vi "Get Array Element Offsets.vi"(8 "error in (no error)":errorcluster, 9 "Max Index":i32=2147483647, 10 "Offset":i32, 11 "JSON":string="[1,2,3]") -> (0 "error out":errorcluster, 1 "Elements":T1[](array[typedef]), 2 "Offset past Array":i32, 4 "Comma Needed for Insert":bool)   [LabVIEW 2024, in "JSONtext.lvlib"]
uses:
  JSONtext.lvlib
  Found Items.ctl
  Parsing State.ctl
  Comma Needed for Insert.ctl
  Advance past Line Ending.vi
  Advance past String.vi
  Advance past Number.vi
  Advance past Array.vi
  Advance past Object.vi
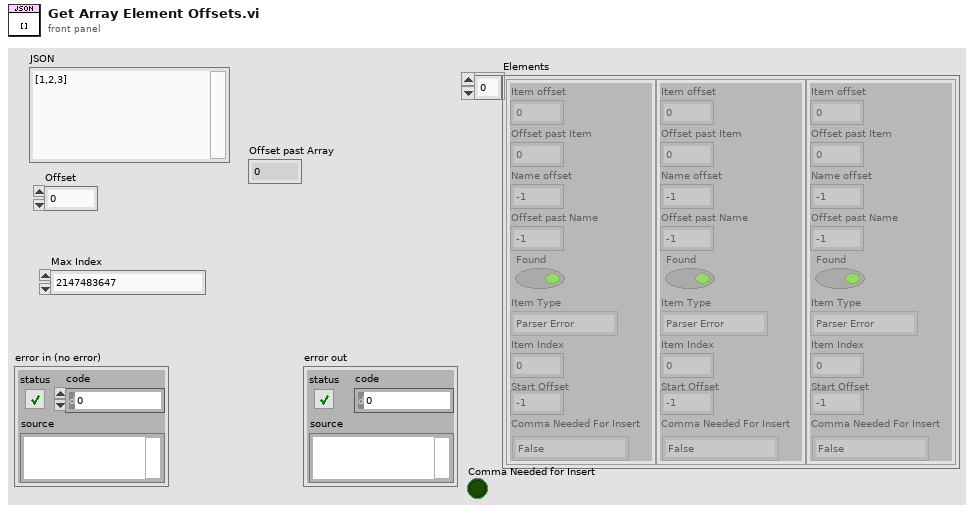
[diagram p1: front panel]
types:
  T1 = typedef "JSONtext.lvlib/Found Items.ctl" = cluster{"Item offset":i32, "Offset past Item":i32, "Name offset":i32, "Offset past Name":i32, "Found":bool, "Item Type":T2, "Item Index":i32, "Start Offset":i32, "Comma Needed For Insert":T3}
  T2 = typedef "JSONtext.lvlib/Parsing State.ctl" = enum16{"Parser Error", "Object", "Array", "String", "Number/Other", "Leading Whitespace", "Object end", "Array end", "Value end"}
  T3 = typedef "JSONtext.lvlib/Comma Needed for Insert.ctl" = enum8{"False", "True", "Following"}
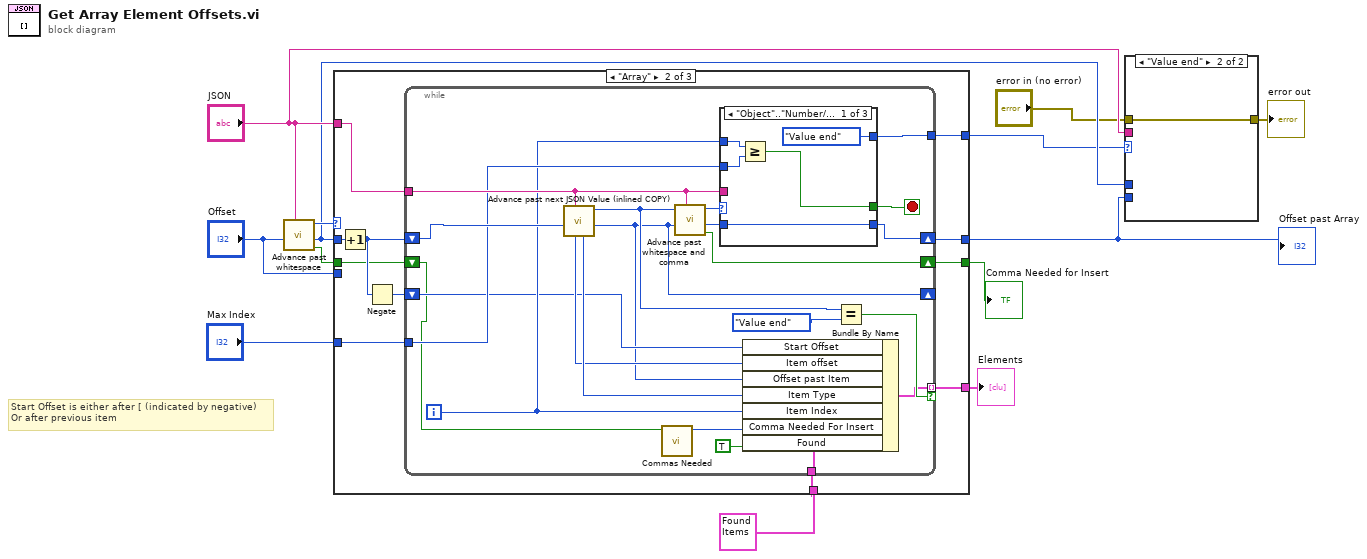
[diagram p0: block diagram]
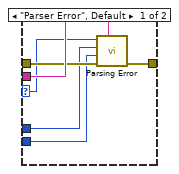
[diagram p2: hidden frame]
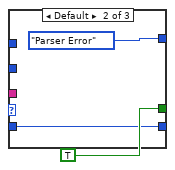
[diagram p4: hidden frame]
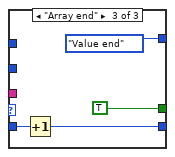
[diagram p5: hidden frame]
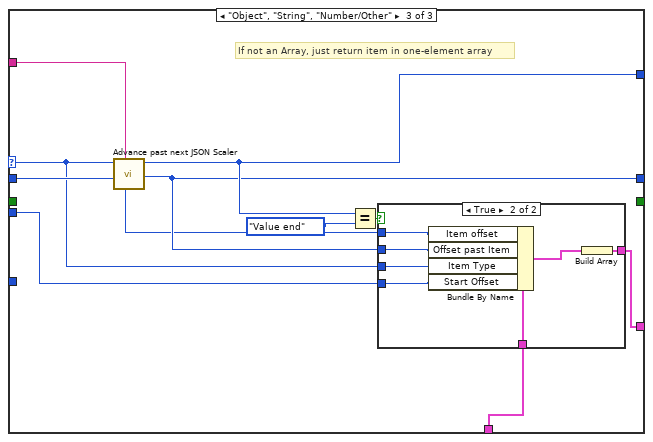
[diagram p6: hidden frame]
diagram:
  # "Start Offset is either after [ (indicated by negative)\nOr after previous item"
  n1 = call "Advance past whitespace.vi"("JSON"="JSON", "Offset"="Offset") -> ("Comma Not Found"=w2:bool, "Offset of first non-whitespace"=w11:i32, "Parser State"=w13:T2)  [unwired: 7 in]
  n2 = case shown="\"Array\"" w13 {
    selector: w13 -> [w15 _ w64]
    tunnel: [w15 w26 w68] -> w7
    tunnel: [w14 w25 w63] -> w10
    tunnel: [_ w24 w66] -> w6
    tunnel: "JSON" -> [_ w23 w69]
    tunnel: w11 -> [w14 w22 w71]
    tunnel: "Max Index" -> [_ w21 _]
    tunnel: T1 {"Item offset"=0, "Offset past Item"=0, "Name offset"=0, "Offset past Name"=0, "Found"=FALSE, "Item Type"=enum."Parser Error", "Item Index"=0, "Start Offset"=0, "Comma Needed For Insert"=enum."False"} -> [_ w20 w65]
    tunnel: "Offset" -> [_ _ w61]
    tunnel: w2 -> [_ w17 _]
    tunnel: [_ w16 _] -> w1
    frame "Parser Error", Default {
    }
    frame "Array" {
      n3 = Increment(x=w22) -> (x+1=w19:i32)
      n4 = Negate(x=w19) -> (-x=w18:i32)
      n5 = while {
        tunnel: w23 -> [w42]
        shift-right: [w45] -> w25
        shift-left: w19 -> [w46]
        tunnel: [w43] -> w26
        tunnel: [w33] -> w24 mode=indexing if=w39
        tunnel: w21 -> [w38]
        tunnel: w20 -> [w37]
        shift-right: [w31] -> _
        shift-left: w18 -> [w32]
        shift-right: [w30] -> w16
        shift-left: w17 -> [w28]
        i -> [w36]
        stop <- w44 stop-if-true
        n6 = call "Advance past next JSON Value (inlined COPY).vi"("JSON"=w42, "Offset"=w46) -> ("Offset"=w31:i32, "State"=w40:T2, "Type"=w35:T2, "Value start"=w34:i32)  [unwired: 5 in, 1 out]
        n7 = call "Commas Needed.vi"("Comma needed"=w28) -> ("Comma Needed For Insert"=w29:T3)  [unwired: 10 in]
        n8 = call "Advance past whitespace and comma.vi"("JSON"=w42, "Offset"=w31, "State in"=w40) -> ("Comma Not Found"=w30:bool, "Offset past match"=w48:i32, "State"=w47:T2)  [unwired: 6 in]
        n9 = case shown="\"Object\"..\"Number/Other\"" w47 {
          tunnel: [w50 TRUE TRUE] -> w44
          tunnel: [Parsing_State."Value end" Parsing_State."Parser Error" Parsing_State."Value end"] -> w43
          tunnel: w48 -> [w53 w54 w58]
          tunnel: [w53 w54 w57] -> w45
          tunnel: w42 -> [_ _ _]
          tunnel: w36 -> [w51 _ _]
          tunnel: w38 -> [w52 _ _]
          frame "Object".."Number/Other" {
            n10 = Greater Or Equal?(x=w51, y=w52) -> (x >= y?=w50:bool)
          }
          frame Default {
          }
          frame "Array end" {
            n11 = Increment(x=w58) -> (x+1=w57:i32)
          }
        }
        n12 = Bundle By Name(cluster=w37, "Start Offset"=w32, "Item offset"=w34, "Offset past Item"=w31, "Item Type"=w35, "Item Index"=w36, "Comma Needed For Insert"=w29, "Found"=TRUE) -> (w33:T1)
        n13 = Equal?(x=w40, y=Parsing_State."Value end") -> (x = y?=w39:bool)
      }
    }
    frame "Object", "String", "Number/Other" {
      # "If not an Array, just return item in one-element array"
      n14 = call "Advance past next JSON Scaler.vi"("JSON"=w69, "Offset"=w71, "Parser State in"=w64) -> ("Offset Past"=w63:i32, "Parser State"=w68:T2, "Value start"=w62:i32)  [unwired: 6 in]
      n15 = Equal?(x=w68, y=Parsing_State."Value end") -> (x = y?=w67:bool)
      n16 = case shown="True" w67 {
        tunnel: [_ w78] -> w66
        tunnel: w65 -> [_ w77]
        tunnel: w64 -> [_ w76]
        tunnel: w63 -> [_ w75]
        tunnel: w62 -> [_ w74]
        tunnel: w61 -> [_ w72]
        frame False {
        }
        frame True {
          n17 = Bundle By Name(cluster=w77, "Item offset"=w74, "Offset past Item"=w75, "Item Type"=w76, "Start Offset"=w72) -> (w73:T1)
          n18 = Build Array(w73) -> (w78:T1[])
        }
      }
    }
  }
  "Offset past Array" <- w10
  "Elements" <- w6
  "Comma Needed for Insert" <- w1
  n19 = case shown="\"Value end\"" w7 {
    selector: w7 -> [w79 _]
    tunnel: "JSON" -> [w84 _]
    tunnel: "error in (no error)" -> [w83 w85]
    tunnel: [w82 w85] -> w9
    tunnel: w11 -> [w81 _]
    tunnel: w10 -> [w80 _]
    frame "Parser Error", Default {
      n20 = call "Parsing Error.vi"("JSON"=w84, "error in (no error)"=w83, "Offset past match"=w80, "Value start"=w81, "State"=w79) -> ("error out"=w82:errorcluster)  [unwired: 6 in]
    }
    frame "Value end" {
    }
  }
  "error out" <- w9
